vi "read.vi"() -> ()   [LabVIEW 2019]
uses:
  <vilib>/Utility/file.llb/Read Delimited Spreadsheet (DBL).vi
panel:
  in  "file path (dialog if empty)":path
  out "size(s)":i32[](array[numeric])
  out "all rows":dbl[][](array[numeric]) format="%0.3f"
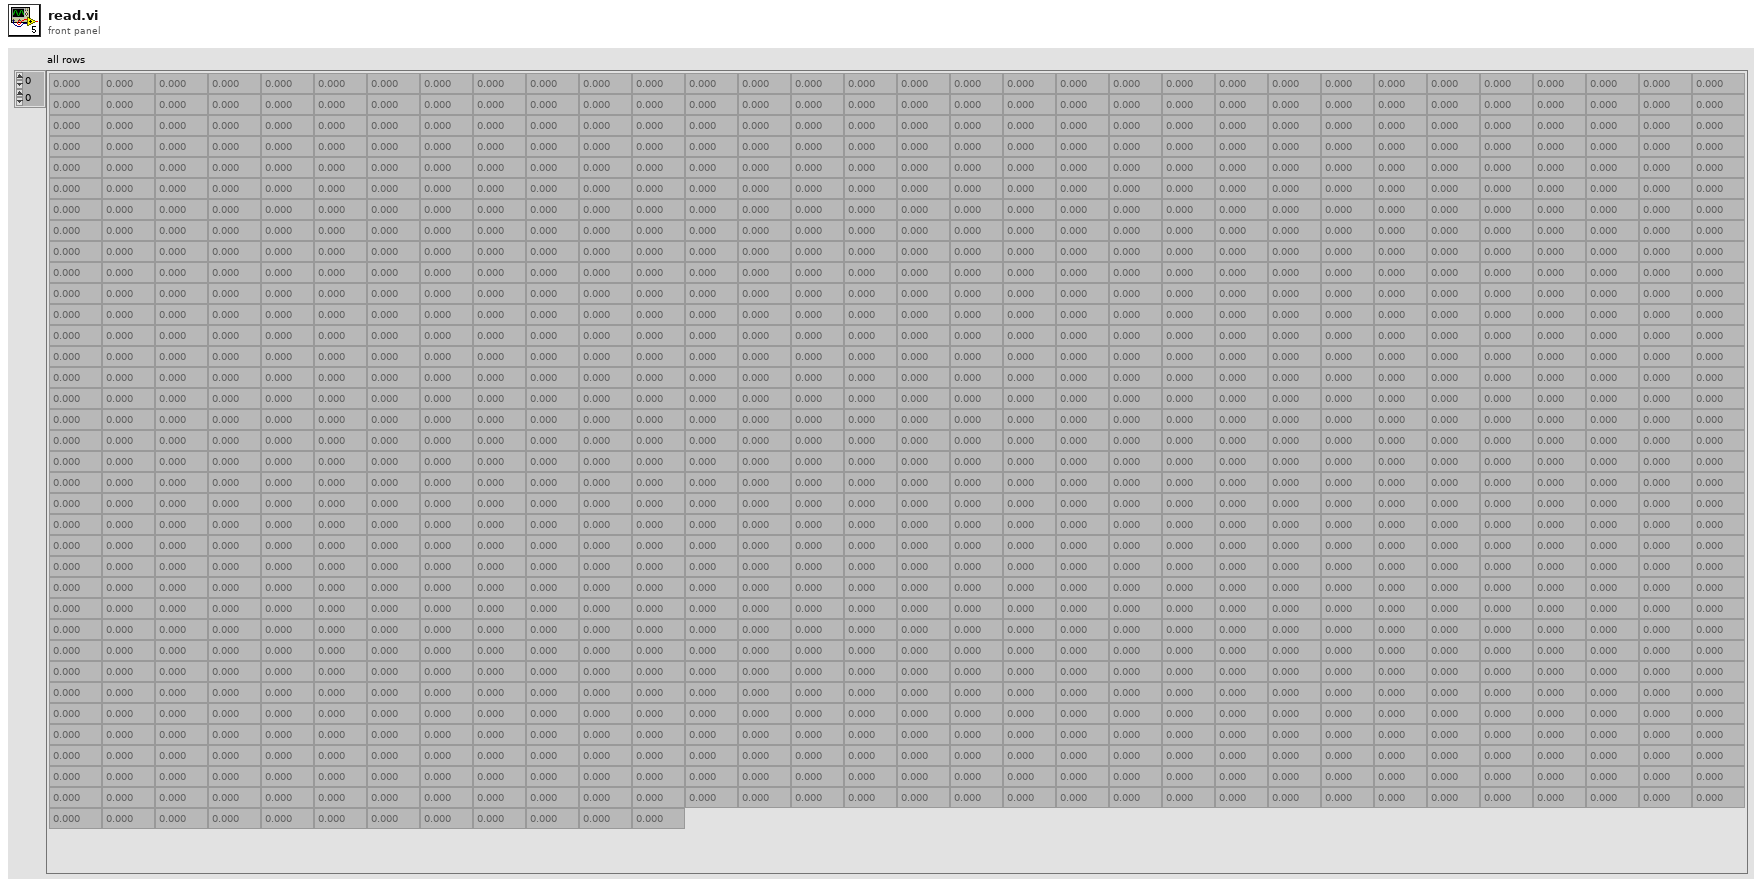
[diagram p1: front panel]
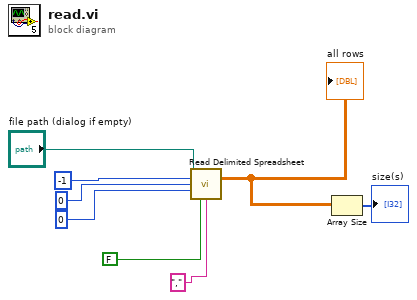
[diagram p0: block diagram]
diagram:
  n1 = call-poly <vilib>:"Read Delimited Spreadsheet.vi"("file path (dialog if empty)"="file path (dialog if empty)", "number of rows (all:-1)"=-1, "start of read offset (chars.:0)"=0, "max characters/row  (no limit:0)"=0, "transpose? (F)"=FALSE ("transpose (no:F)"), "delimiter (\\t)"=",") -> ("all rows"=w7:dbl[][])  [unwired: 4 in, 5 out]
  "all rows" <- w7
  n2 = Array Size(array=w7) -> (size(s)=→"size(s)":i32[])
